vi "BooleanMode.vi"(1 "5.3.0 How Check Light  2":bool) -> (0 "5.3.0 How Check Light":bool)   [LabVIEW 2010]
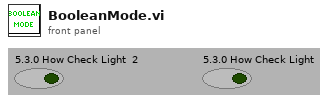
[diagram p1: front panel]
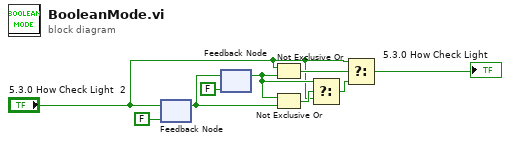
[diagram p0: block diagram]
diagram:
  n1 = feedback #1(FALSE) -> (w3:bool)
  n2 = feedback-in #1("5.3.0 How Check Light  2") -> ()
  n3 = feedback #2(FALSE) -> (w5:bool)
  n4 = feedback-in #2(w3) -> ()
  n5 = Not Exclusive Or(1:w5, 2:"5.3.0 How Check Light  2") -> (0:w7:bool)
  n6 = Not Exclusive Or(1:w3, 2:w5) -> (0:w4:bool)
  n7 = Select(t=w5, s=w4, f="5.3.0 How Check Light  2") -> (s? t:f=w6:bool)
  n8 = Select(t="5.3.0 How Check Light  2", s=w7, f=w6) -> (s? t:f=→"5.3.0 How Check Light":bool)
